vi "Config.vi"(8 "error in (no error)":errorcluster, 10 "Setting":variant, 11 "CompactRIO in":refnum<class "CompactRIO.lvclass">) -> (0 "error out":errorcluster, 3 "CompactRIO out":refnum<class "CompactRIO.lvclass">)   [LabVIEW 2025, in "FPGA.lvlib" / "CompactRIO.lvclass"]
uses:
  CompactRIO.lvclass
  C:/Users/Public/Documents/Sandia National Labs/TSS Plugin/CEF.lvlibp/Node/CEF_Node.lvclass
  FPGA Channel/FPGA Channel.lvclass
  FPGA Channel configuration/FPGA Channel configuration.lvclass
  C:/Users/Public/Documents/Sandia National Labs/TSS Plugin/Abstract Engine.lvlibp/Plugin/Abstract/Channel configuration/Channel configuration.lvclass
  CompactRIO.lvclass/CompactRIO.ctl
  Users/Public/Documents/Sandia National Labs/TSS Plugin/CEF.lvlibp/Node/ReadChildren.vi
  Users/Public/Documents/Sandia National Labs/TSS Plugin/Abstract Engine.lvlibp/Plugin/Abstract/Channel configuration/Read Channel Setting.vi
  Users/Public/Documents/Sandia National Labs/TSS Plugin/CEF.lvlibp/Node/CEF_Node.lvclass
  Users/Public/Documents/Sandia National Labs/TSS Plugin/CEF.lvlibp/serializable configuration/CEF_serializable configuration.lvclass
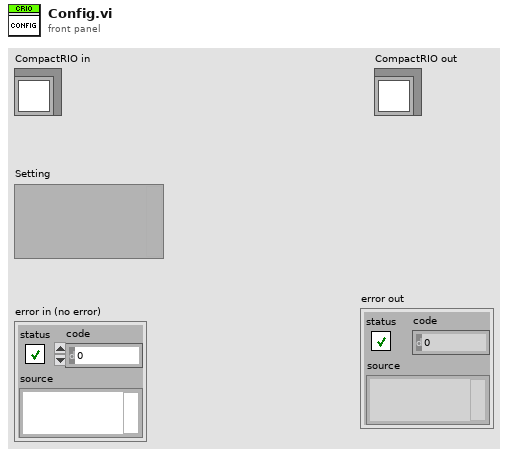
[diagram p1: front panel]
types:
  T1 = cluster{"Address":string, "SW Alias":string, "Description":string, "Enabled":bool, "Node Class":string}
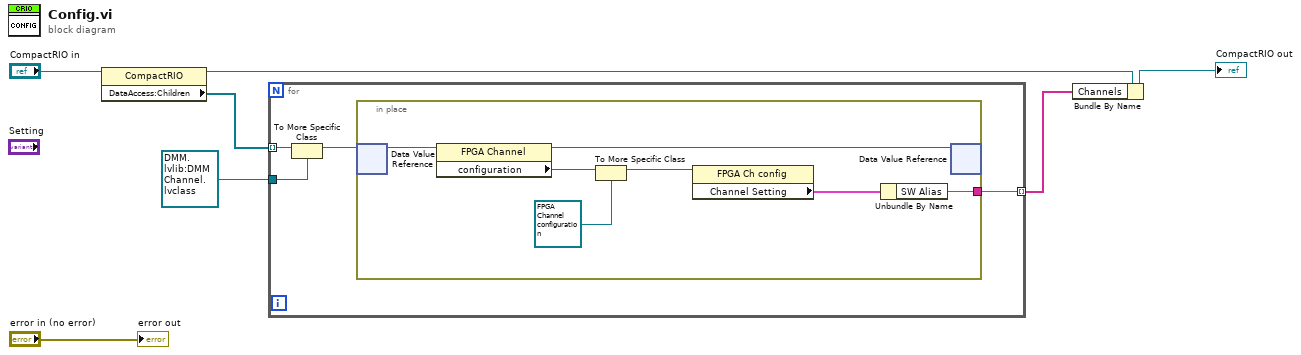
[diagram p0: block diagram]
diagram:
  n1 = property class="CompactRIO"(reference="CompactRIO in") -> (reference out=w5:refnum<class "CompactRIO.lvclass">, "DataAccess:Children"=w4:refnum<data-value>[])  [unwired: 1 in, 1 out]
  n2 = for {
    tunnel: w4 -> [w11] mode=indexing
    tunnel: [w9] -> w3 mode=indexing
    tunnel: refnum<data-value> refnum ("data value reference") -> [w8]
    n3 = To More Specific Class(target class=w8, reference=w11) -> (specific class reference=w10:refnum<data-value>)  [unwired: 1 in, 1 out]
    n4 = in-place {
      in-place-border: [w14] -> w9
      n5 = in-place-dvr #1(w10) -> (w18:refnum<class "FPGA Channel.lvclass">)  [unwired: 1 out]
      n6 = property class="FPGA Channel"(reference=w18) -> (reference out=w17:refnum<class "FPGA Channel.lvclass">, "configuration"=w16:refnum<class "CEF_serializable configuration.lvclass">)  [unwired: 1 in, 1 out]
      n7 = To More Specific Class(target class=refnum<class "FPGA Channel configuration.lvclass"> refnum ("Plugin.lvlib:Device Channel configuration.lvclass"), reference=w16) -> (specific class reference=w15:refnum<class "FPGA Channel configuration.lvclass">)  [unwired: 1 in, 1 out]
      n8 = property class="FPGA Ch config"(reference=w15) -> ("Channel Setting"=w12:T1)  [unwired: 1 in, 2 out]
      n9 = Unbundle By Name(w12) -> ("SW Alias"=w14:string)
      n10 = in-place-dvr #1(w17) -> ()  [unwired: 2 out]
    }
  }
  n11 = Bundle By Name(cluster=w5, "Channels"=w3) -> (→"CompactRIO out":refnum<class "CompactRIO.lvclass">)
  "error out" <- "error in (no error)"
